vi "FATEK_HexToString.vi"(10 "字符个数":i32=6, 11 "数组":u16[](array[numeric]) format="%04xH") -> (3 "STRING":string[](array[string]))   [LabVIEW 2016, in "PLC.lvlib"]
uses:
  PLC.lvlib
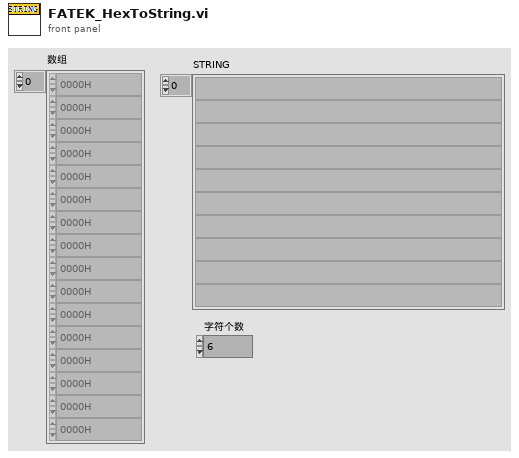
[diagram p1: front panel]
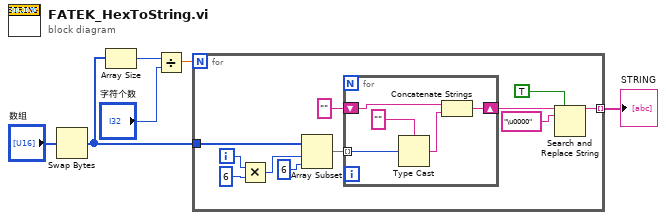
[diagram p0: block diagram]
diagram:
  n1 = Swap Bytes(anything="数组") -> (byte swapped=w1:u16[])
  n2 = Array Size(array=w1) -> (size(s)=w6:i32)
  n3 = Divide(x=w6, y="字符个数") -> (x/y=w4:dbl)
  n4 = for {
    N: w4 -> [_]
    tunnel: w1 -> [w17]
    tunnel: [w9] -> w3 mode=indexing
    i -> [w16]
    n5 = Multiply(x=w16, y=6) -> (x*y=w13:i32)
    n6 = Array Subset(array=w17, index=w13, length=6 ("索引")) -> (w11:u16[])
    n7 = for {
      shift-right: [w22] -> w10
      shift-left: "" -> [w19]
      tunnel: w11 -> [w21] mode=indexing
      n8 = Type Cast(type="", x=w21) -> (*(type *) &x=w18:string)
      n9 = Concatenate Strings(w19, w18) -> (w22:string)
    }
    n10 = Search and Replace String(replace all?=TRUE ("替换全部？(F)"), input string=w10, search string="\u0000" ("搜索字符串")) -> (result string=w9:string)  [unwired: 5 in, 3 out]
  }
  "STRING" <- w3
